vi "Messaging EnQ Single.vi"(5 "Command":string, 6 "@Front?":bool, 7 "Data":variant, 8 "error in (no error)":errorcluster) -> (0 "error out":errorcluster)   [LabVIEW 2019, in "GUI.lvlib"]
doc: "Enqueue a single <b>Command</b> with variant <b>Data</b>. Optionally choose if you want the element <b>@Front</b> of the Q."
uses:
  GUI.lvlib
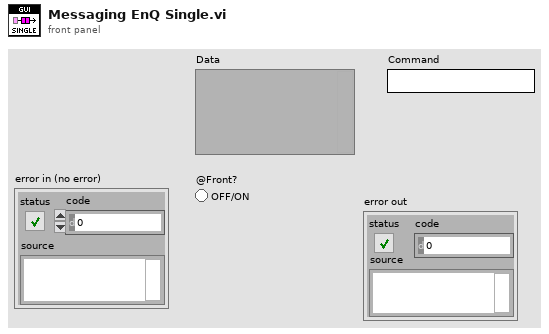
[diagram p1: front panel]
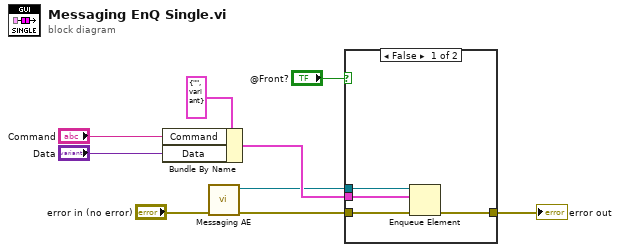
[diagram p0: block diagram]
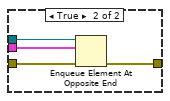
[diagram p2: hidden frame]
diagram:
  n1 = Bundle By Name(cluster=cluster{"Command":string, "Data":variant} {"Command"="", "Data"=variant} ("Message Data"), "Command"="Command", "Data"="Data") -> (w6:cluster{"Command":string, "Data":variant})
  n2 = call "Messaging AE.vi"("Error In"="error in (no error)") -> ("Error Out"=w3:errorcluster, "queue out"=w2:refnum<queue>)  [unwired: 9 in]
  n3 = case shown="False" "@Front?" {
    tunnel: w6 -> [w13 w17]
    tunnel: w2 -> [w12 w16]
    tunnel: [w11 w15] -> w9
    tunnel: w3 -> [w10 w14]
    frame False {
      n4 = Enqueue Element(queue=w12, element=w13, error in (no error)=w10) -> (error out=w11:errorcluster)  [unwired: 1 in, 2 out]
    }
    frame True {
      n5 = Enqueue Element At Opposite End(queue=w16, element=w17, error in (no error)=w14) -> (error out=w15:errorcluster)  [unwired: 1 in, 2 out]
    }
  }
  "error out" <- w9
